vi "GetZeroOffset.vi"(8 "error in":errorcluster, 10 "Device Key In":string, 11 "PM Cmds In":refnum<k24>) -> (0 "error out":errorcluster, 1 "Zero Offset":string, 2 "Device Key Out":string, 3 "PM Cmds Out":refnum<k24>)   [LabVIEW 2010]
uses:
  C:/Code/Apps/Utilities/PM2935/PMWinApp/PM_Installer/Master/Samples/1918 - 2936 Family/LabVIEW/LabVIEW 2010/PowerMeterCommands.dll
  PowerMeterCommands.dll
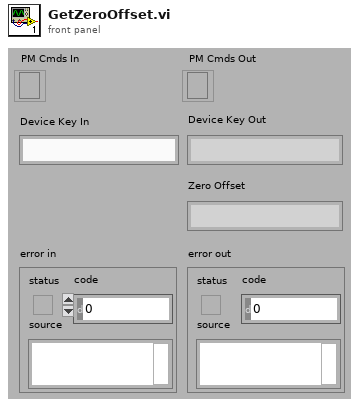
[diagram p1: front panel]
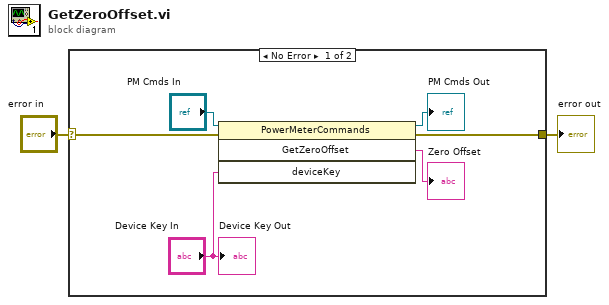
[diagram p0: block diagram]
diagram:
  n1 = case shown="No Error" "error in" {
    selector: "error in" -> [w5 w9]
    tunnel: [w4 w9] -> w1
    frame No Error {
      n2 = invoke class="PowerMeterCommands" method="GetZeroOffset"(reference="PM Cmds In", error in=w5, "deviceKey"="Device Key In") -> (reference out=→"PM Cmds Out":refnum<k24>, error out=w4:errorcluster, "GetZeroOffset"=→"Zero Offset":string)  [unwired: 1 in, 1 out]
      "Device Key Out" <- "Device Key In"
    }
    frame Error {
    }
  }
  "error out" <- w1
